vi "Define Test Suite.vi"(8 "error in (no error)":errorcluster, 9 "Report Path":path, 10 "Interactive":bool, 11 "Label (VI Title)":string) -> (0 "error out":errorcluster, 3 "Test Suite":refnum<class "Test Suite.lvclass">)   [LabVIEW 2009, in "Caraya.lvlib" / "Test Suite.lvclass"]
doc: "Registers the calling VI as a test suite. If Interactive is True, the interactive user interface is opened when the test suite is executed. If the Report Path is set, a report file will be generated with the test results.\n\n--\nCopyright © 2015 JKI All rights reserved.\n\nAuthor: Tomi Maila <tomi.maila@jki.net>\n\nThis library is provided \"AS IS\" ,WITHOUT WARRANTIES OR\nCONDITIONS OF ANY KIND, either express or implied.\n\nJKI -- jki.net"
uses:
  Test Suite.lvclass
  Test Assert Factory/Test Assert Factory.lvclass
  Test Report.Default/Test Report.Default.lvclass
  Assert Factory/Assert Factory.lvclass
  Test Suite.lvclass/Test Suite.ctl
  Test Manager/Test Manager.lvclass
  Caraya.lvlib
  Assert Factory Manager/Assert Factory Manager.lvclass
panel:
  # "Copyright © 2015 JKI All rights reserved.\n\nAuthor: Tomi Maila <tomi.maila@jki.net>\n\nThis library is provided \"AS IS\" ,WITHOUT WARRANTIES OR\nCONDITIONS OF ANY KIND, either express or implied.\n\nJKI -- jki.net"
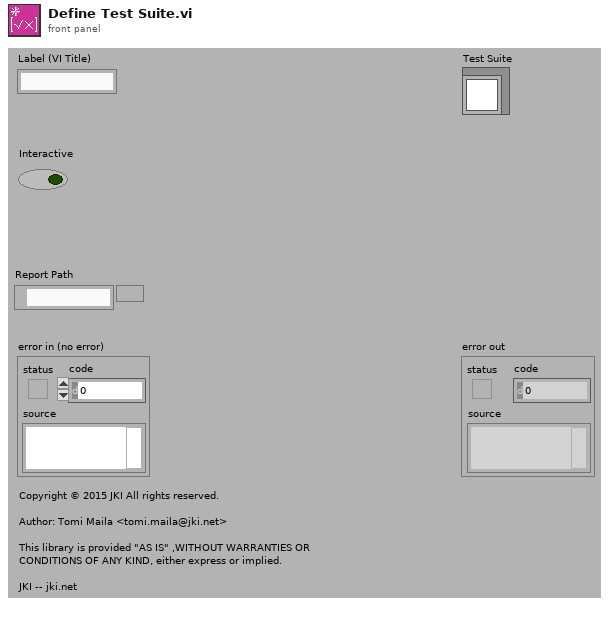
[diagram p1: front panel]
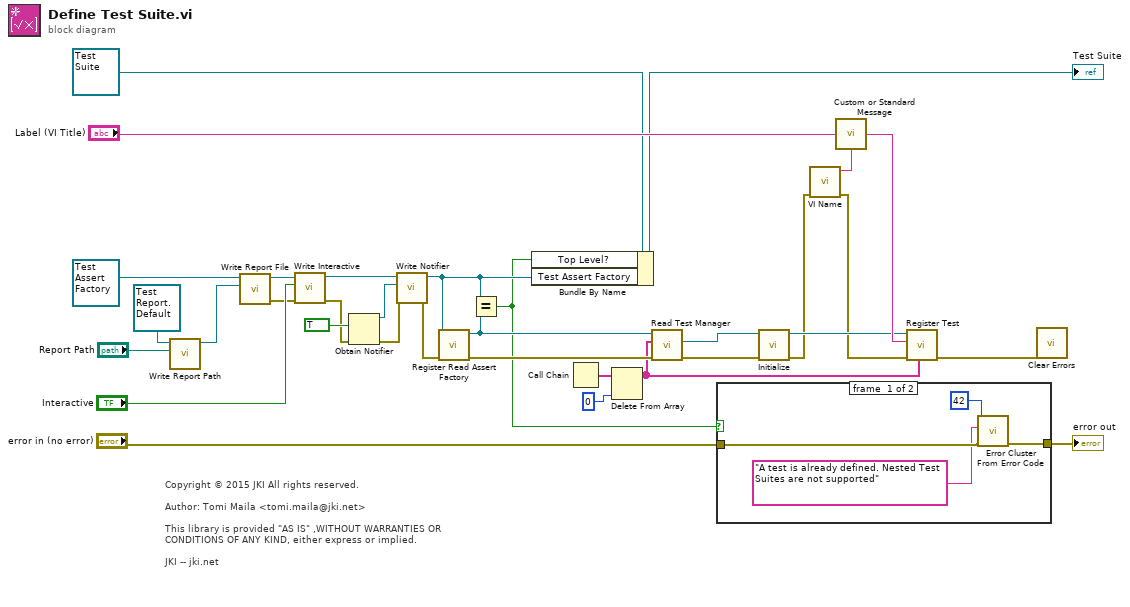
[diagram p0: block diagram]
diagram:
  # "Copyright © 2015 JKI All rights reserved.\n\nAuthor: Tomi Maila <tomi.maila@jki.net>\n\nThis library is provided \"AS IS\" ,WITHOUT WARRANTIES OR\nCONDITIONS OF ANY KIND, either express or implied.\n\nJKI -- jki.net"
  n1 = call "Write Report Path.vi"("Report Path"="Report Path", "Test Report.Default in"=refnum<class "Test Report.Default.lvclass"> refnum ("Caraya.lvlib:Test Report.Default.lvclass")) -> ("Test Report.Default out"=w1:refnum<class "Test Report.Default.lvclass">)  [unwired: 9 in]
  n2 = call "Write Report File.vi"("Test Report"=w1, "Test Assert Factory in"=refnum<class "Test Assert Factory.lvclass"> refnum ("Caraya.lvlib:Test Assert Factory.lvclass")) -> ("error out"=w28:errorcluster, "Test Assert Factory out"=w30:refnum<class "Test Assert Factory.lvclass">)  [unwired: 8 in]
  n3 = call "Write Interactive.vi"("error in (no error)"=w28, "Interactive"="Interactive", "Test Assert Factory in"=w30) -> ("error out"=w22:errorcluster, "Test Assert Factory out"=w25:refnum<class "Test Assert Factory.lvclass">)  [unwired: 7 in]
  n4 = Obtain Notifier(notification data type=TRUE, error in (no error)=w22) -> (notifier out=w20:refnum<notifier>, error out=w21:errorcluster)  [unwired: 2 in, 1 out]
  n5 = call "Write Notifier.vi"("error in (no error)"=w21, "notifier"=w20, "Test Assert Factory in"=w25) -> ("error out"=w26:errorcluster, "Test Assert Factory out"=w9:refnum<class "Test Assert Factory.lvclass">)  [unwired: 7 in]
  n6 = call "Register Read Assert Factory.vi"("error in (no error)"=w26, "Assert Factory"=w9) -> ("error out"=w32:errorcluster, "Assert Factory"=w8:refnum<class "Assert Factory.lvclass">)  [unwired: 8 in]
  n7 = Equal?(x=w9, y=w8) -> (x = y?=w5:bool)
  n8 = Bundle By Name(cluster=refnum<class "Test Suite.lvclass"> refnum ("Test Suite"), "Top Level?"=w5, "Test Assert Factory"=w9) -> (→"Test Suite":refnum<class "Test Suite.lvclass">)
  n9 = Call Chain() -> (call chain=w11:string[])
  n10 = Delete From Array(array=w11, index=0) -> (array with subset deleted=w10:string[])  [unwired: 1 in, 1 out]
  n11 = call-dynamic "Read Test Manager.vi"("error in (no error)"=w32, "VI Call Chain"=w10, "Assert Factory in"=w8) -> ("error out"=w16:errorcluster, "Test Manager"=w4:refnum<class "Test Manager.lvclass">)  [unwired: 6 in, 1 out]
  n12 = case shown="False" w5 {
    tunnel: [w37 w38] -> w7
    tunnel: "error in (no error)" -> [w36 w38]
    frame #0 {
      n13 = call <vilib>:"Error Cluster From Error Code.vi"("error in (no error)"=w36, "error message (\"\")"="A test is already defined. Nested Test Suites are not supported" ("error message (\"\")"), "error code (0)"=42) -> ("error out"=w37:errorcluster)  [unwired: 6 in]
    }
    frame #1 {
    }
  }
  "error out" <- w7
  n14 = call-dynamic "Initialize.vi"("error in (no error)"=w16, "Test Manager in"=w4) -> ("error out"=w15:errorcluster, "Test Manager out"=w17:refnum<class "Test Manager.lvclass">)  [unwired: 8 in]
  n15 = call "VI Name.vi"("error in (no error)"=w15) -> ("error out"=w14:errorcluster, "VI Name"=w19:string)  [unwired: 9 in]
  n16 = call "Custom or Standard Message.vi"("Custom Message"="Label (VI Title)", "Standard Message"=w19) -> ("Message"=w18:string)
  n17 = call-dynamic "Register Test.vi"("Call Chain"=w10, "error in (no error)"=w14, "Name"=w18, "Test Manager in"=w17) -> ("error out"=w13:errorcluster)  [unwired: 6 in, 1 out]
  n18 = call <vilib>:"Clear Errors.vi"("error in (no error)"=w13) -> ()  [unwired: 6 in, 1 out]
